vi "Dispatch Rx Plugin.vi"(8 "error in (no error)":errorcluster, 10 "Plugin in":refnum<class "Plugin.lvclass">, 11 "Dispatcher Interface in":refnum<class "Dispatcher Interface.lvclass">) -> (0 "error out":errorcluster, 2 "Plugin out":refnum<class "Plugin.lvclass">, 3 "Dispatcher Interface out":refnum<class "Dispatcher Interface.lvclass">)   [LabVIEW 2017, in "DSF Core.lvlib" / "Dispatcher Interface.lvclass"]
uses:
  Interfaces/Dispatcher/Dispatcher Interface.lvclass
  Plugin/Plugin.lvclass
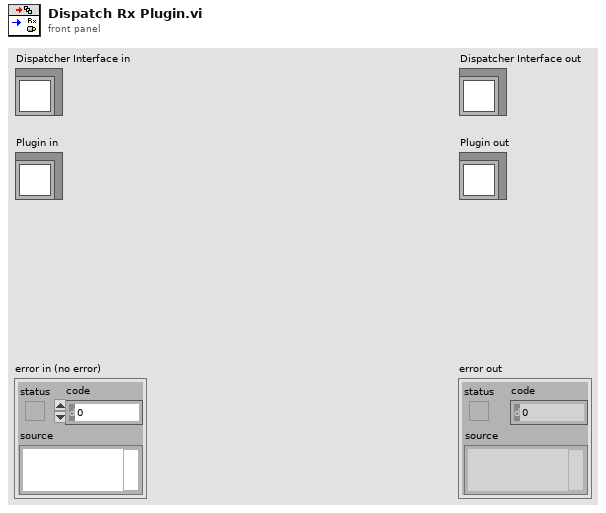
[diagram p1: front panel]
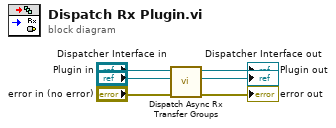
[diagram p0: block diagram]
diagram:
  n1 = call "Dispatch Async Rx Transfer Groups.vi"("error in (no error)"="error in (no error)", "Dispatcher Interface in"="Dispatcher Interface in", "Plugin in"="Plugin in") -> ("error out"=→"error out":errorcluster, "Dispatcher Interface out"=→"Dispatcher Interface out":refnum<class "Dispatcher Interface.lvclass">, "Plugin out"=→"Plugin out":refnum<class "Plugin.lvclass">)  [unwired: 6 in]
